vi "Cont.vi"(10 "Compiler Settings":T1={"Python Path"=path "", "Main File"="makesequence.py", "Meta File"="makesequence.py", "Aux File"="makesequence.py", "Pre File"="metascript.txt"}, 11 "MetaorMain":enum16{"Meta", "Main"}(ring)) -> ()   [LabVIEW 2019]
uses:
  PulseCompiler/CompilerSettings.ctl
panel:
  in  "stop":bool
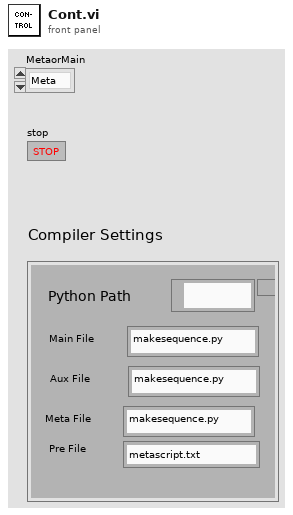
[diagram p1: front panel]
types:
  T1 = typedef "CompilerSettings.ctl" = cluster{"Python Path":path, "Main File":string, "Meta File":string, "Aux File":string, "Pre File":string}
  T2 = cluster{"command":string, "steps":i32, "runs":i32}[]
  T3 = typedef "PulseControl.ctl" = cluster{"FPGA Code":cluster{"Times":u32[], "Pulses":u64[], "Counts":u8[], "Triggers":u8[], "AOs":u8[], "# of runs":i32, "Line trig?":bool, "time photons?":bool}, "AWG pulses array":variant[], "Params":T4}
  T4 = typedef "Params.ctl" = cluster{"steps":i16, "runs":i16, "comment":string, "mathematica":string, "calib":i8, "logmsg":string, "ndets":i16}
  T5 = cluster{"readout":u32[][], "kinetic series data":i32[][][][], "camera dim":cluster{i32, i32, i32, i32}}
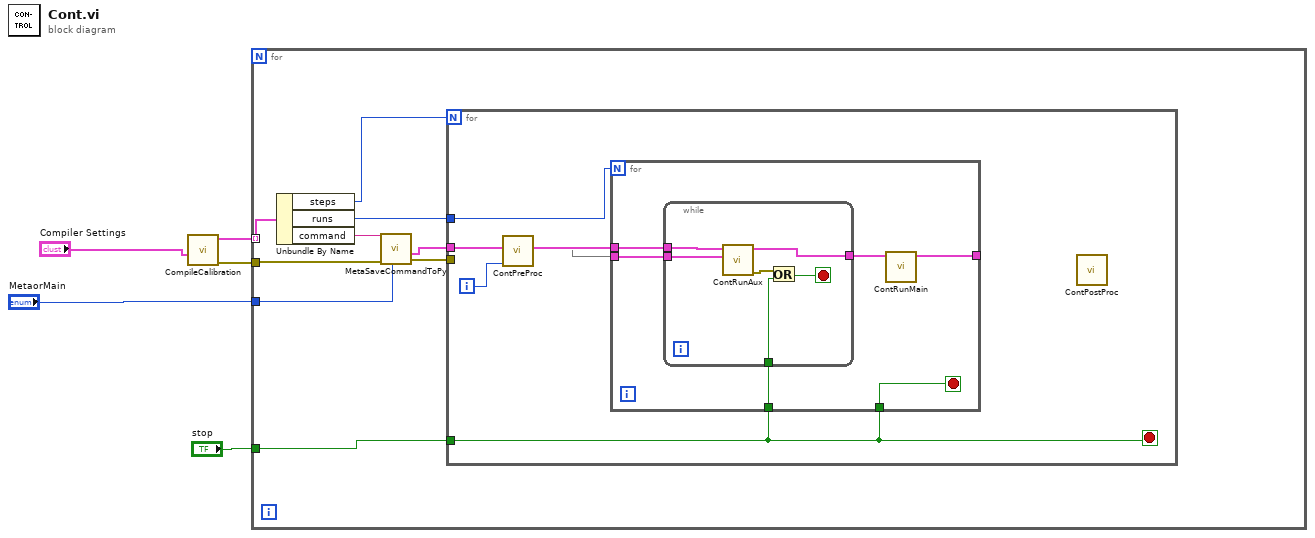
[diagram p0: block diagram]
diagram:
  n1 = call "CompileCalibration.vi"("Compiler Settings"="Compiler Settings") -> ("error out"=w4:errorcluster, "Exp out"=w3:T2)  [unwired: 8 in, 1 out]
  n2 = for {
    tunnel: "stop" -> [w14]
    tunnel: w4 -> [w8]
    tunnel: w3 -> [w13] mode=indexing
    tunnel: "MetaorMain" -> [w7]
    n3 = Unbundle By Name(w13) -> ("steps"=w12:i32, "runs"=w11:i32, "command"=w10:string)
    n4 = call "MetaSaveCommandToPy.vi"("MetaorMain"=w7, "error in"=w8, "command"=w10) -> ("error out"=w9:errorcluster, "Compiler Settings Out"=w6:T1)  [unwired: 7 in]
    n5 = for {
      N: w12 -> [_]
      tunnel: w14 -> [w19]
      tunnel: w9 -> [_]
      tunnel: w11 -> [w16]
      tunnel: w6 -> [w15]
      i -> [w20]
      stop <- w19 stop-if-true
      n6 = call "ContPreProc.vi"("error in (no error)"=w20, "Compiler Settings"=w15) -> (2:w17, "Main pulse seq"=w18:T3)  [unwired: 4 in, 4 out]
      n7 = for {
        N: w16 -> [_]
        tunnel: w19 -> [w25]
        tunnel: w19 -> [w24]
        tunnel: [w23] -> _
        tunnel: w18 -> [w22]
        tunnel: w17 -> [w21]
        stop <- w25 stop-if-true
        n8 = while {
          tunnel: [w31] -> w26
          tunnel: w24 -> [w29]
          tunnel: w22 -> [w28]
          tunnel: w21 -> [w27]
          stop <- w32 stop-if-true
          n9 = call "ContRunAux.vi"("Aux pulse in"=w27, "Main Pulse In"=w28) -> ("error out"=w30:errorcluster, "Main Pulse Out"=w31:T3)  [unwired: 7 in, 1 out]
          n10 = Or(x=w30, y=w29) -> (x .or. y?=w32:bool)
        }
        n11 = call "ContRunMain.vi"("Main Pulse In"=w26) -> ("readout"=w23:T5)  [unwired: 8 in, 2 out]
      }
      n12 = call "ContPostProc.vi"() -> ()  [unwired: 11 in, 1 out]
    }
  }
